vi "parameter setup.vi"() -> ()   [LabVIEW 2018]
uses:
  4f91c110-3135-4dd2-83ce-6201250ee320.vi
panel:
  out "f2":dbl
  out "f1":dbl
  out "f3":dbl
  in  "阻抗管内径(mm):":dbl
  in  "传声器3到样品距离x3(mm)：":dbl
  in  "传声器2到样品距离x2(mm)：":dbl
  in  "传声器1到样品距离x1(mm)：":dbl
  in  "保存":T1
  in  "待测样品面积S(mm^2)：":dbl
  in  "传声器4到样品距离L(mm)：":dbl
  in  "mic4灵敏度(V/Pa)：":dbl
  in  "管中温度(℃)：":dbl
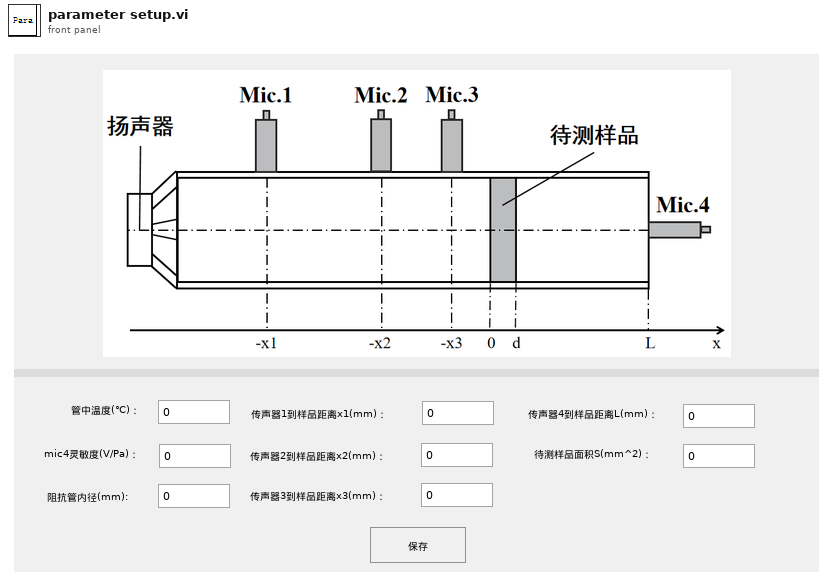
[diagram p1: front panel]
types:
  T1 = typedef "布尔控件.ctl" = bool
  T2 = cluster{"管中温度：":dbl, "阻抗管内径d[mm]：":dbl, "传声器4到样品距离L[mm]：":dbl, "待测样品面积S[mm^2]：":dbl, "mic4灵敏度(V/Pa)：":dbl, "传声器1到样品距离x1[mm]：":dbl, "传声器1到样品距离x2[mm]：":dbl, "传声器1到样品距离x3[mm]：":dbl, "f1":dbl, "f2":dbl, "f3":dbl}
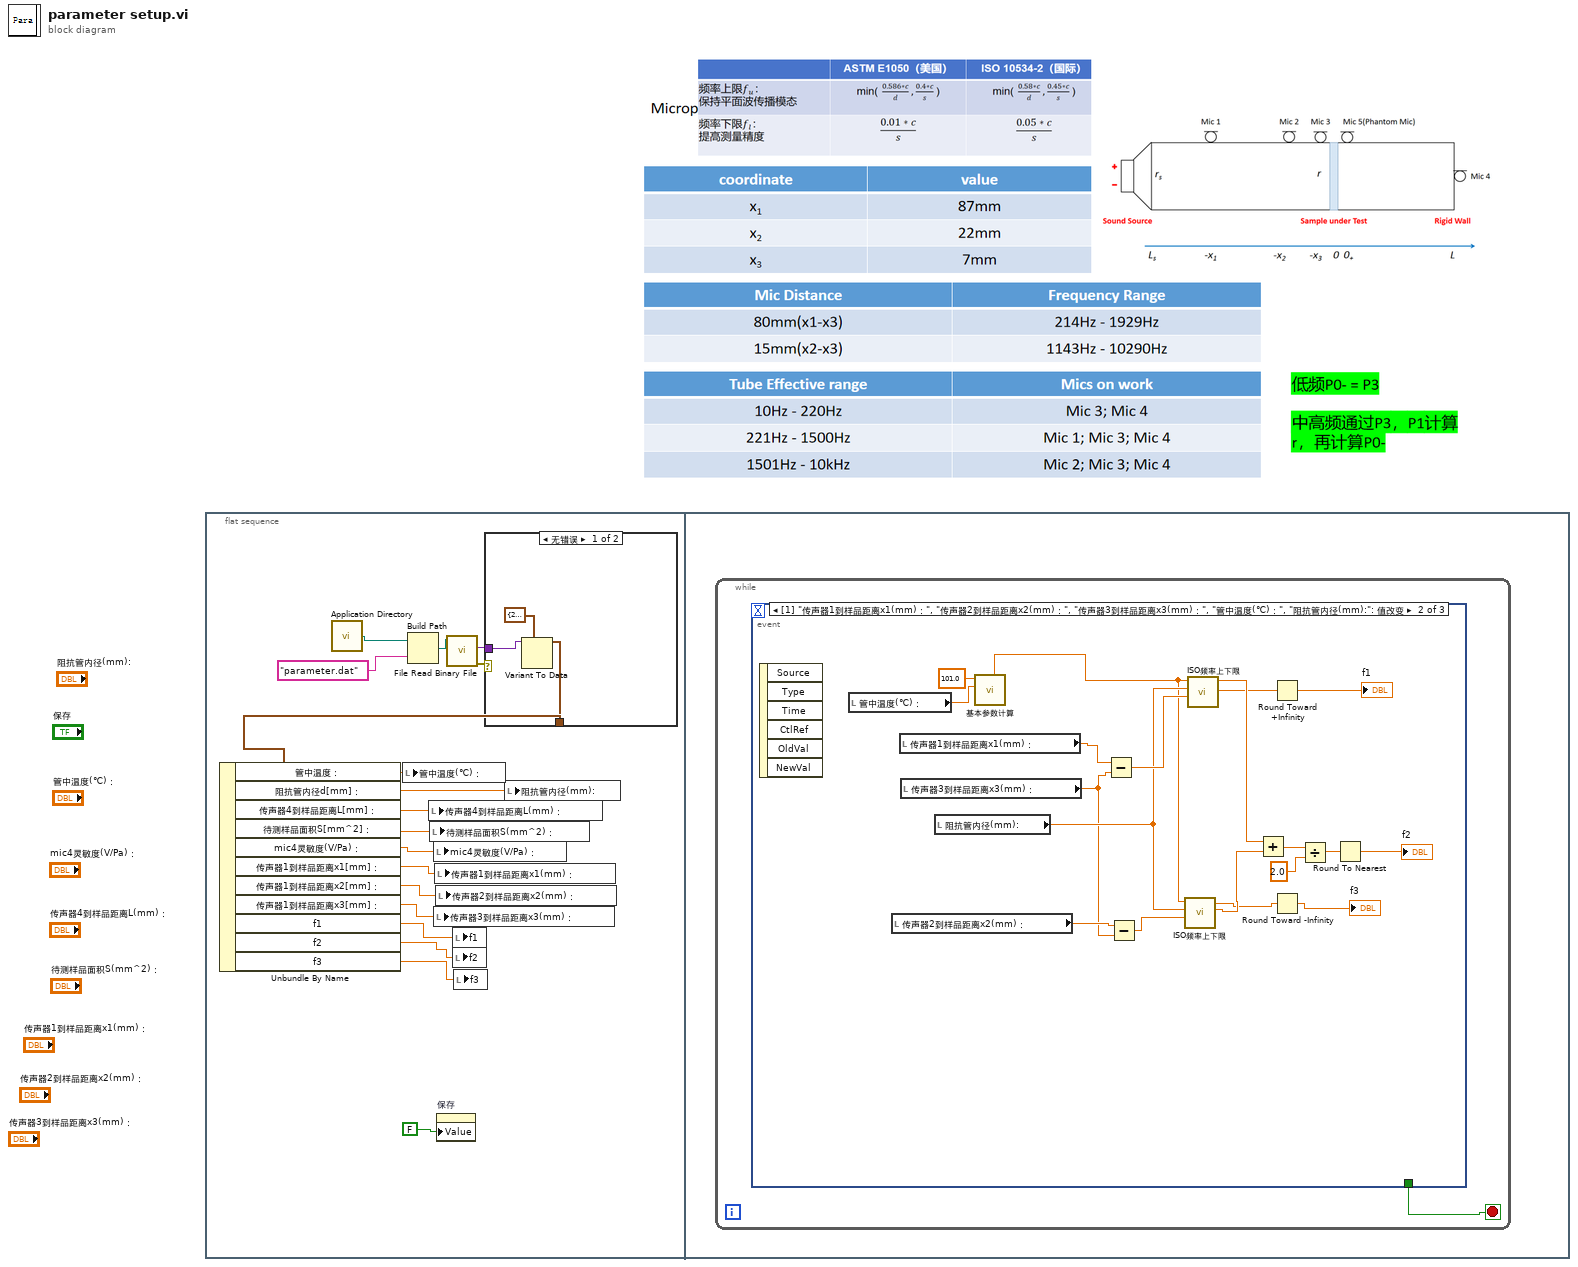
[diagram p0: block diagram]
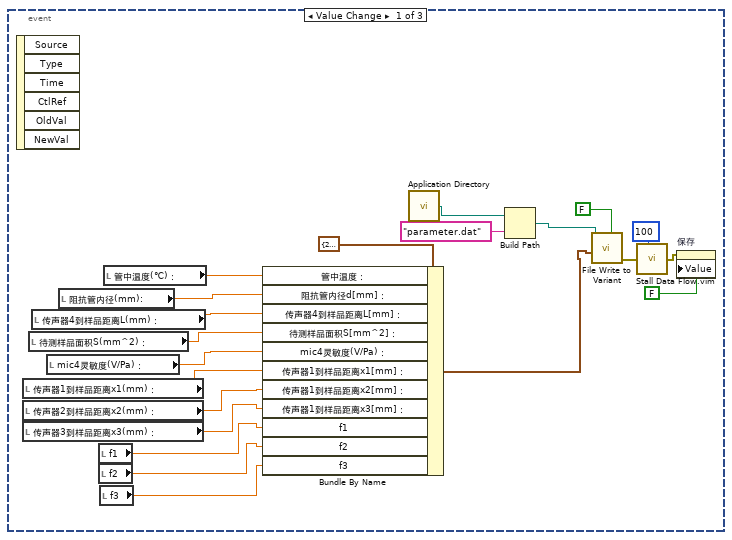
[diagram p3: hidden frame]
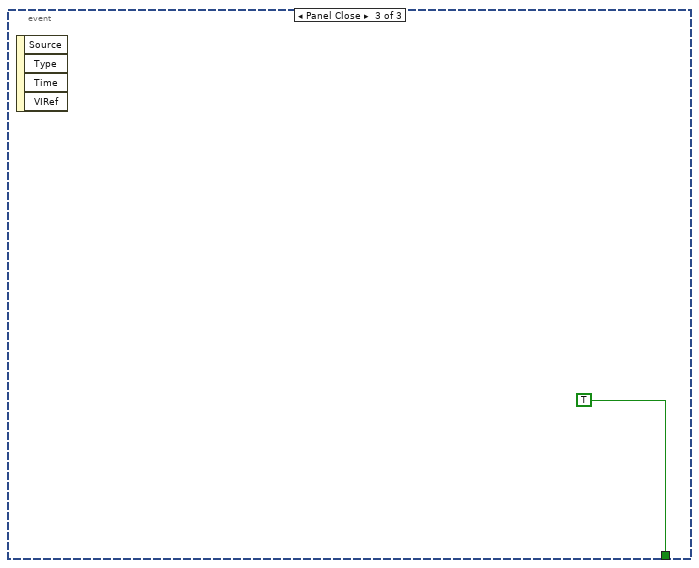
[diagram p4: hidden frame]
diagram:
  n1 = flat-sequence {
    frame #0 {
      n2 = call <vilib>:"Application Directory.vi"() -> ("Application Directory"=w8:path)
      n3 = Build Path(base path=w8, name or relative path="parameter.dat" ("名称或相对路径")) -> (appended path=w17:path)
      n4 = property on="保存" class="Bool (严格)"("Value"=T1 FALSE ("计算频率上下限")) -> ()  [unwired: 2 in, 2 out]
      n5 = call "File Read Binary File.vi"("file path"=w17) -> ("error Output"=w9:errorcluster, "Variant Output"=w16:variant)  [unwired: 8 in, 1 out]
      n6 = case shown="无错误" w9 {
        tunnel: w16 -> [w21 _]
        tunnel: [w20 _] -> w15
        frame No Error {
          n7 = Variant To Data(type=T2 {"管中温度："=22.0, "阻抗管内径d[mm]："=0.2, "传声器4到样品距离L[mm]："=0.025, "待测样品面积S[mm^2]："=0.15, "mic4灵敏度(V/Pa)："=0.0, "传声器1到样品距离x1[mm]："=0.0, "传声器1到样品距离x2[mm]："=0.0, "传声器1到样品距离x3[mm]："=0.0, "f1"=0.0, "f2"=0.0, "f3"=0.0}, Variant=w21) -> (data=w20:T2)  [unwired: 1 in, 1 out]
        }
        frame Error {
        }
      }
      n8 = Unbundle By Name(w15) -> ("管中温度："=w14:dbl, "阻抗管内径d[mm]："=w13:dbl, "传声器4到样品距离L[mm]："=w12:dbl, "待测样品面积S[mm^2]："=w11:dbl, "mic4灵敏度(V/Pa)："=w7:dbl, "传声器1到样品距离x1[mm]："=w6:dbl, "传声器1到样品距离x2[mm]："=w5:dbl, "传声器1到样品距离x3[mm]："=w4:dbl, "f1"=w3:dbl, "f2"=w2:dbl, "f3"=w1:dbl)
      n9 = local write "管中温度(℃)："(w14) -> ()
      n10 = local write "传声器4到样品距离L(mm)："(w12) -> ()
      n11 = local write "待测样品面积S(mm^2)："(w11) -> ()
      n12 = local write "mic4灵敏度(V/Pa)："(w7) -> ()
      n13 = local write "传声器3到样品距离x3(mm)："(w4) -> ()
      n14 = local write "传声器1到样品距离x1(mm)："(w6) -> ()
      n15 = local write "传声器2到样品距离x2(mm)："(w5) -> ()
      n16 = local write "f1"(w3) -> ()
      n17 = local write "f2"(w2) -> ()
      n18 = local write "f3"(w1) -> ()
      n19 = local write "阻抗管内径(mm):"(w13) -> ()
    }
    frame #1 {
      n20 = while {
        stop <- w22 stop-if-true
        n21 = event shown="[1] \"传声器1到样品距离x1(mm)：\", \"传声器2到样品距离x2(mm)：\", \"传声器3到样品距离x3(mm)：\", \"管中温度(℃)：\", \"阻抗管内径(mm):\": 值改变" {
          selector: _ -> [_ _ _]
          dyn-events: _ -> [_ _ _]
          timeout: _ -> [_ _ _]
          tunnel: [_ _ TRUE] -> w22
          event Value Change {
            n22 = event-data() -> ()  [unwired: 1 in, 6 out]
            n23 = local read "传声器1到样品距离x1(mm)："() -> (w33:dbl)
            n24 = local read "传声器2到样品距离x2(mm)："() -> (w27:dbl)
            n25 = local read "传声器3到样品距离x3(mm)："() -> (w26:dbl)
            n26 = local read "待测样品面积S(mm^2)："() -> (w39:dbl)
            n27 = local read "传声器4到样品距离L(mm)："() -> (w40:dbl)
            n28 = local read "mic4灵敏度(V/Pa)："() -> (w34:dbl)
            n29 = local read "阻抗管内径(mm):"() -> (w38:dbl)
            n30 = local read "f1"() -> (w25:dbl)
            n31 = local read "f2"() -> (w24:dbl)
            n32 = local read "f3"() -> (w23:dbl)
            n33 = local read "管中温度(℃)："() -> (w41:dbl)
            n34 = Bundle By Name(cluster=T2 {"管中温度："=22.0, "阻抗管内径d[mm]："=0.2, "传声器4到样品距离L[mm]："=0.025, "待测样品面积S[mm^2]："=0.15, "mic4灵敏度(V/Pa)："=0.0, "传声器1到样品距离x1[mm]："=0.0, "传声器1到样品距离x2[mm]："=0.0, "传声器1到样品距离x3[mm]："=0.0, "f1"=0.0, "f2"=0.0, "f3"=0.0}, "管中温度："=w41, "阻抗管内径d[mm]："=w38, "传声器4到样品距离L[mm]："=w40, "待测样品面积S[mm^2]："=w39, "mic4灵敏度(V/Pa)："=w34, "传声器1到样品距离x1[mm]："=w33, "传声器1到样品距离x2[mm]："=w27, "传声器1到样品距离x3[mm]："=w26, "f1"=w25, "f2"=w24, "f3"=w23) -> (w37:T2)
            n35 = call <vilib>:"Application Directory.vi"() -> ("Application Directory"=w28:path)
            n36 = Build Path(base path=w28, name or relative path="parameter.dat" ("名称或相对路径")) -> (appended path=w42:path)
            n37 = call "File Write to Variant.vi"("替换提示"=FALSE, "Input Data"=w37, "Path to Write"=w42) -> ("error out"=w32:errorcluster)  [unwired: 4 in, 4 out]
            n38 = call "Stall Data Flow.vim"("value in"=w32, "milliseconds to wait"=u32 100) -> ("value out"=w30:errorcluster)  [unwired: 1 out]
            n39 = property on="保存" class="Bool (严格)"(error in=w30, "Value"=T1 FALSE ("保存")) -> ()  [unwired: 1 in, 2 out]
          }
          event "传声器1到样品距离x1(mm)：", "传声器2到样品距离x2(mm)：", "传声器3到样品距离x3(mm)：", "管中温度(℃)：", "阻抗管内径(mm):": Value Change {
            n40 = event-data() -> ()  [unwired: 1 in, 6 out]
            n41 = local read "管中温度(℃)："() -> (w60:dbl)
            n42 = local read "传声器2到样品距离x2(mm)："() -> (w45:dbl)
            n43 = local read "传声器1到样品距离x1(mm)："() -> (w62:dbl)
            n44 = local read "传声器3到样品距离x3(mm)："() -> (w44:dbl)
            n45 = local read "阻抗管内径(mm):"() -> (w57:dbl)
            n46 = call "基本参数计算.vi"("temp实际摄氏温度"=w60, "atm/kPa"=101.0) -> ("考虑温度实际声速c0"=w56:dbl)  [unwired: 7 in, 2 out]
            n47 = Subtract(x=w62, y=w44) -> (x-y=w59:dbl)
            n48 = Subtract(x=w45, y=w44) -> (x-y=w58:dbl)
            n49 = call "ISO频率上下限.vi"("麦克风间距s[mm]"=w58, "管直径d[mm]"=w57, "声速c"=w56) -> ("频率下限fL"=w55:dbl, "频率上限fu"=w49:dbl)  [unwired: 7 in]
            n50 = call "ISO频率上下限.vi"("麦克风间距s[mm]"=w59, "管直径d[mm]"=w57, "声速c"=w56) -> ("频率下限fL"=w51:dbl, "频率上限fu"=w54:dbl)  [unwired: 7 in]
            n51 = Add(x=w54, y=w55) -> (x+y=w53:dbl)
            n52 = Round Toward +Infinity(x=w51) -> (ceil(x): smallest int >= x=→"f1":dbl)
            n53 = Round Toward -Infinity(1:w49) -> (0:→"f3":dbl)
            n54 = Divide(x=w53, y=2.0) -> (x/y=w47:dbl)
            n55 = Round To Nearest(number=w47) -> (nearest integer value=→"f2":dbl)
          }
          event Panel Close {
            n56 = event-data() -> ()  [unwired: 1 in, 4 out]
          }
        }
      }
    }
  }
